vi "Divide Quaternions.vi"   [LabVIEW 2017, in "NI_Kinematics.lvlib"]
doc: "Computes the <B>quotient</B> of two quaternions or a quaternion and a scalar number. Wire data to the <B>y</B> input to determine the polymorphic instance to use or manually select the instance."
uses:
  <vilib>/robotics/Kinematics/NI_Kinematics.lvlib
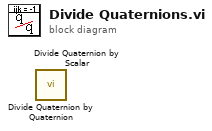
[diagram p0: block diagram]
diagram:
  n1 = call <vilib>:"Divide Quaternion by Quaternion.vi"() -> ()  [unwired: 2 in, 1 out]
  n2 = call <vilib>:"Divide Quaternion by Scalar.vi"() -> ()  [unwired: 2 in, 1 out]
